vi "BLM_IgnoreAlarms.vi"() -> ()   [LabVIEW 2019]
panel:
  in  "Ignore Alarms":bool
  # "THIS VI is used by BLM Status and BLM Init"
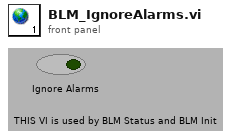
[diagram p1: front panel]
diagram:
